vi "Dashboard Main.vi"() -> ()   [LabVIEW 2012]
uses:
  <vilib>/Utility/config.llb/Read Key (String).vi
  <vilib>/Utility/config.llb/Read Key (I32).vi
  <vilib>/Utility/config.llb/NI_LVConfig.lvlib
panel:
  in  "Y Coord":dbl=140.0
  in  "X Coord":dbl=200.0
  in  "Size":u16(ring)=1 items=["640x480", "320x240", "160x120"]
  in  "Compression":i32=30
  out "Mbps":dbl format="%#.1g"
  in  "Enable":bool=TRUE
  out "fps":dbl format="%#.1g"
  out "Camera Image":T1(plugin-control)
  out "Camera Image 2":T1(plugin-control)
  out "Camera IP 2":string
  out "Camera IP":string
  out "fps 2":dbl format="%#.1g"
  out "Mbps 2":dbl format="%#.1g"
  in  "Enable 2":bool=TRUE
  in  "Frame Rate":i32=15
  out "Battery Value":dbl(slide) scale=0.0..14.0 scale format="%#_2e"
  out "Battery":sgl(graph)
  out "Robot IP":string
  out "Mode":T2(ring)=enum."Auto Disabled"
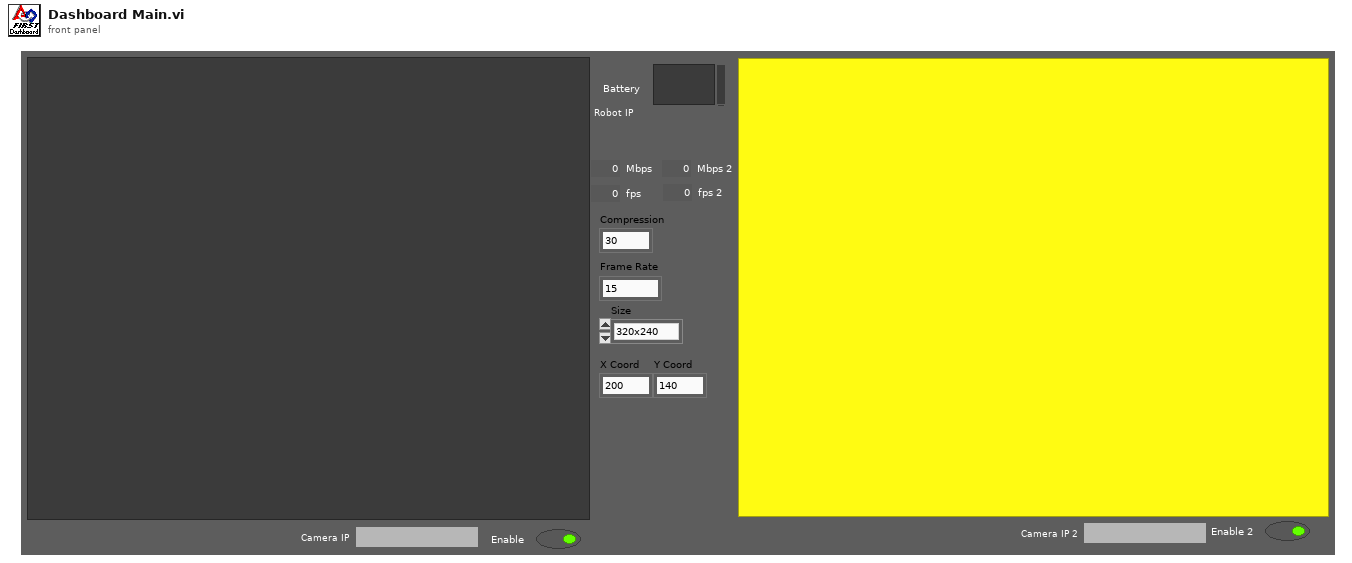
[diagram p1: front panel]
types:
  T1 = typedef "IMAQ Image.ctl" = refnum<image>
  T2 = enum8{"Tele-Op Disabled", "Tele-Op Enabled", "Auto Disabled", "Auto Enabled", "Test Disabled", "Test Enabled", ""}
  T3 = typedef "Image Type" = u32
  T4 = typedef "NI_LVConfig.lvlib/Config Data RefNum.ctl" = refnum<k1>
  T5 = cluster{"Competition mode":bool, "Robot Link":bool, "Autonomous":bool, "Enabled":bool, "E-Stop":bool, "Simulated":bool, "TestMode":bool, "Docked Window":bool}
  T6 = typedef "LVRectTypeDef.ctl" = cluster{"Left":i16, "Top":i16, "Right":i16, "Bottom":i16}
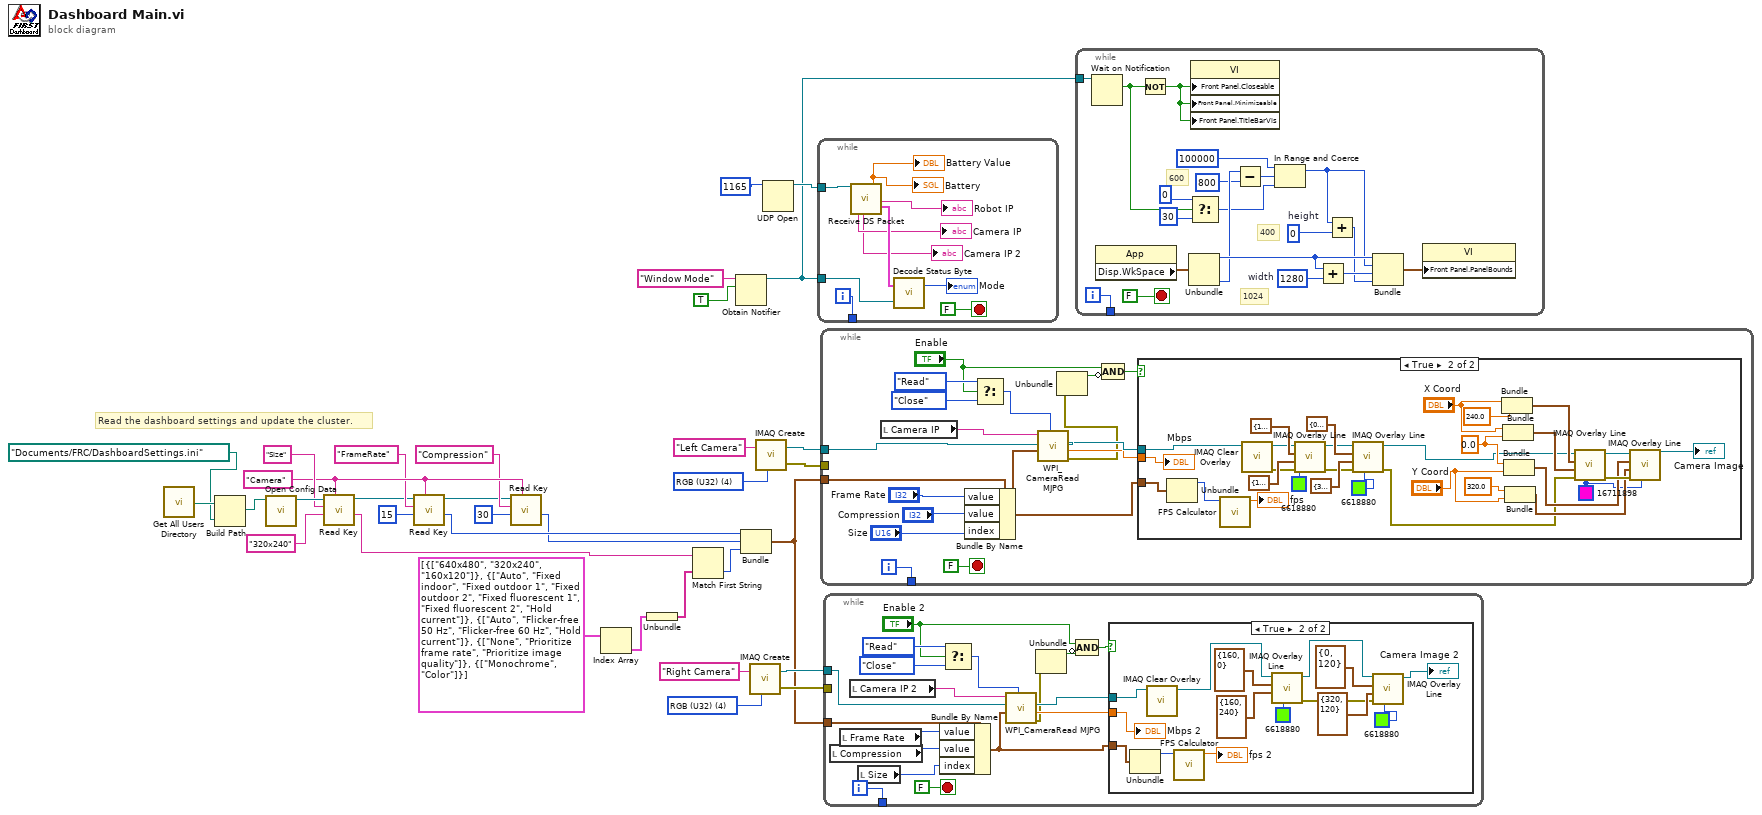
[diagram p0: block diagram]
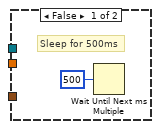
[diagram p2: hidden frame]
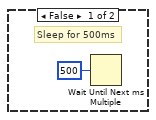
[diagram p3: hidden frame]
diagram:
  w4 = T3 4 items=["Grayscale (U8)", "Grayscale (I16)", "Grayscale (SGL)", "Complex (CSG)", "RGB (U32)", "HSL (U32)", "RGB (U64)"] ("Image Type")
  w20 = "Camera"
  w32 = T3 4 items=["Grayscale (U8)", "Grayscale (I16)", "Grayscale (SGL)", "Complex (CSG)", "RGB (U32)", "HSL (U32)", "RGB (U64)"] ("Image Type")
  # "Read the dashboard settings and update the cluster."
  n1 = call "Get All Users Directory.vi"() -> ("All User Path"=w25:path)
  n2 = Build Path(base path=w25, name or relative path=path "Documents/FRC/DashboardSettings.ini") -> (appended path=w24:path)
  n3 = call <vilib>:"Open Config Data.vi"("configuration file path"=w24) -> ("refnum"=w23:T4)  [unwired: 8 in, 2 out]
  n4 = call-poly <vilib>:"Read Key.vi"("section"=w20, "default value"="320x240", "key"="Size", "refnum"=w23) -> ("value"=w10:string, "refnum out"=w7:T4)  [unwired: 2 in, 4 out]
  n5 = call-poly <vilib>:"Read Key.vi"("section"=w20, "default value"=15, "key"="FrameRate", "refnum"=w7) -> ("value"=w15:i32, "refnum out"=w6:T4)  [unwired: 1 in, 5 out]
  n6 = call-poly <vilib>:"Read Key.vi"("section"=w20, "default value"=30, "key"="Compression", "refnum"=w6) -> ("value"=w14:i32)  [unwired: 1 in, 6 out]
  n7 = Index Array(array=cluster{string[]}[] [{["640x480", "320x240", "160x120"]}, {["Auto", "Fixed indoor", "Fixed outdoor 1", "Fixed outdoor 2", "Fixed fluorescent 1", "Fixed fluorescent 2", "Hold current"]}, {["Auto", "Flicker-free 50 Hz", "Flicker-free 60 Hz", "Hold current"]}, {["None", "Prioritize frame rate", "Prioritize image quality"]}, {["Monochrome", "Color"]}]) -> (element=w13:cluster{string[]})  [unwired: 1 in]
  n8 = Unbundle(w13) -> (w11:string[])
  n9 = Match First String(2:w11, 3:w10) -> (0:w9:i32)  [unwired: 1 out]
  n10 = Obtain Notifier(name (unnamed)="Window Mode", notification data type=TRUE) -> (notifier out=w26:refnum<notifier>)  [unwired: 2 in, 2 out]
  n11 = Bundle("value"=w15, "value"=w14, "index"=w9) -> (w1:cluster{"value":i32, "value":i32, "index":i32})  [unwired: 1 out]
  n12 = call "IMAQ Create"("Image Name"="Right Camera", "Image Type"=w4) -> ("New Image"=w3:T1, "error out"=w2:errorcluster)  [unwired: 2 in, 1 out]
  n13 = call "IMAQ Create"("Image Name"="Left Camera", "Image Type"=w32) -> ("New Image"=w30:T1, "error out"=w29:errorcluster)  [unwired: 2 in, 1 out]
  n14 = UDP Open(11:u16 1165 ("port")) -> (port=w33:refnum<k16>)  [unwired: 2 in, 4 out]
  n15 = while {
    tunnel: w33 -> [w42]
    tunnel: w26 -> [w40]
    tunnel: [w37] -> _
    i -> [w37]
    stop <- FALSE stop-if-true
    n16 = call "Receive DS Packet.vi"("Recv Socket"=w42) -> ("Camera IP Address"=→"Camera IP":string, "Camera IP Address 2"=→"Camera IP 2":string, "Battery"=→"Battery" →"Battery Value":sgl, "Robot IP Address"=→"Robot IP":string, "Status"=w43:T5)  [unwired: 8 in, 6 out]
    n17 = call "Decode Status Byte.vi"("Window Mode Notifier"=w40, "Status"=w43) -> ("Mode"=→"Mode":T2)  [unwired: 1 out]
  }
  n18 = while {
    tunnel: w30 -> [w59]
    tunnel: w29 -> [_]
    tunnel: [w61] -> _
    tunnel: w1 -> [w47]
    i -> [w61]
    stop <- FALSE stop-if-true
    n19 = local read "Camera IP"() -> (w60:string)
    n20 = Bundle By Name(cluster=w47, "value"="Frame Rate", "value"="Compression", "index"="Size") -> (w48:cluster{"value":i32, "value":i32, "index":i32})
    n21 = Select(t=enum16{"Read", "Reopen", "Close"}."Read" ("Operation"), s="Enable", f=enum16{"Read", "Reopen", "Close"}."Close" ("Operation")) -> (s? t:f=w54:enum16{"Read", "Reopen", "Close"})
    n22 = call <vilib>:"WPI_CameraRead MJPG.vi"("Operation"=w54, "Camera Settings"=w48, "Image"=w59, "address"=w60) -> ("error out"=w53:errorcluster, "Bandwidth (kbps)"=w57:dbl, "Image Out"=w58:T1)  [unwired: 5 in]
    n23 = Unbundle(w53) -> ("status"=w51:bool)  [unwired: 2 out]
    n24 = Compound Arithmetic op=AND("Enable", invert w51) -> (w50:bool)
    n25 = case shown="True" w50 {
      tunnel: w48 -> [_ w90]
      tunnel: w58 -> [_ w93]
      tunnel: w57 -> [_ w92]
      frame False {
        # "Sleep for 500ms"
        n26 = Wait Until Next ms Multiple(millisecond multiple=u32 500) -> ()  [unwired: 1 out]
      }
      frame True {
        w64 = u32 16711898 ("Color")
        w77 = 0.0 ("element")
        n27 = Unbundle(w90) -> ("value"=w81:i32)  [unwired: 2 out]
        n28 = call "FPS Calculator.vi"("Average Count"=w81) -> ("fps"=→"fps":dbl)  [unwired: 10 in]
        n29 = call "IMAQ Clear Overlay"("Image"=w93) -> ("error out"=w79:errorcluster, "Image Out"=w82:T1)  [unwired: 2 in, 7 out]
        n30 = call "IMAQ Overlay Line"("Color"=u32 6618880, "error in (no error)"=w79, "End Point"=cluster{"X":i32, "Y":i32} {"X"=160, "Y"=240}, "Start Point"=cluster{"X":i32, "Y":i32} {"X"=160, "Y"=0}, "Image"=w82) -> ("error out"=w87:errorcluster, "Image Out"=w86:T1)  [unwired: 5 in]
        n31 = call "IMAQ Overlay Line"("Color"=u32 6618880, "error in (no error)"=w87, "End Point"=cluster{"X":i32, "Y":i32} {"X"=320, "Y"=120}, "Start Point"=cluster{"X":i32, "Y":i32} {"X"=0, "Y"=120}, "Image"=w86) -> ("error out"=w65:errorcluster, "Image Out"=w66:T1)  [unwired: 5 in]
        n32 = Bundle("X Coord"="X Coord", "element"=240.0) -> (w70:cluster{"X Coord":dbl, "element":dbl})  [unwired: 1 in]
        n33 = Bundle("X Coord"="X Coord", "element"=w77) -> (w69:cluster{"X Coord":dbl, "element":dbl})  [unwired: 1 in]
        n34 = Bundle("element"=w77, "Y Coord"="Y Coord") -> (w68:cluster{"element":dbl, "Y Coord":dbl})  [unwired: 1 in]
        n35 = Bundle("element"=320.0, "Y Coord"="Y Coord") -> (w67:cluster{"element":dbl, "Y Coord":dbl})  [unwired: 1 in]
        n36 = call "IMAQ Overlay Line"("Color"=w64, "error in (no error)"=w65, "End Point"=w69, "Start Point"=w70, "Image"=w66) -> ("error out"=w72:errorcluster, "Image Out"=w73:T1)  [unwired: 5 in]
        n37 = call "IMAQ Overlay Line"("Color"=w64, "error in (no error)"=w72, "End Point"=w67, "Start Point"=w68, "Image"=w73) -> ("Image Out"=→"Camera Image":T1)  [unwired: 5 in, 1 out]
        "Mbps" <- w92
      }
    }
  }
  n38 = while {
    tunnel: w3 -> [w108]
    tunnel: [w110] -> _
    tunnel: w2 -> [_]
    tunnel: w1 -> [w96]
    i -> [w110]
    stop <- FALSE stop-if-true
    n39 = local read "Compression"() -> (w95:i32)
    n40 = local read "Frame Rate"() -> (w98:i32)
    n41 = local read "Camera IP 2"() -> (w109:string)
    n42 = local read "Size"() -> (w94:u16)
    n43 = Bundle By Name(cluster=w96, "value"=w98, "value"=w95, "index"=w94) -> (w97:cluster{"value":i32, "value":i32, "index":i32})
    n44 = Select(t=enum16{"Read", "Reopen", "Close"}."Read" ("Operation"), s="Enable 2", f=enum16{"Read", "Reopen", "Close"}."Close" ("Operation")) -> (s? t:f=w103:enum16{"Read", "Reopen", "Close"})
    n45 = call <vilib>:"WPI_CameraRead MJPG.vi"("Operation"=w103, "Camera Settings"=w97, "Image"=w108, "address"=w109) -> ("error out"=w102:errorcluster, "Bandwidth (kbps)"=w106:dbl, "Image Out"=w107:T1)  [unwired: 5 in]
    n46 = Unbundle(w102) -> ("status"=w100:bool)  [unwired: 2 out]
    n47 = Compound Arithmetic op=AND("Enable 2", invert w100) -> (w99:bool)
    n48 = case shown="True" w99 {
      tunnel: w97 -> [_ w124]
      tunnel: w107 -> [_ w127]
      tunnel: w106 -> [_ w126]
      frame False {
        # "Sleep for 500ms"
        n49 = Wait Until Next ms Multiple(millisecond multiple=u32 500) -> ()  [unwired: 1 out]
      }
      frame True {
        n50 = Unbundle(w124) -> ("value"=w123:i32)  [unwired: 2 out]
        n51 = call "IMAQ Clear Overlay"("Image"=w127) -> ("Image Out"=w114:T1)  [unwired: 2 in, 8 out]
        n52 = call "FPS Calculator.vi"("Average Count"=w123) -> ("fps"=→"fps 2":dbl)  [unwired: 10 in]
        n53 = call "IMAQ Overlay Line"("Color"=u32 6618880, "End Point"=cluster{"X":i32, "Y":i32} {"X"=160, "Y"=240}, "Start Point"=cluster{"X":i32, "Y":i32} {"X"=160, "Y"=0}, "Image"=w114) -> ("error out"=w120:errorcluster, "Image Out"=w119:T1)  [unwired: 6 in]
        n54 = call "IMAQ Overlay Line"("Color"=u32 6618880, "error in (no error)"=w120, "End Point"=cluster{"X":i32, "Y":i32} {"X"=320, "Y"=120}, "Start Point"=cluster{"X":i32, "Y":i32} {"X"=0, "Y"=120}, "Image"=w119) -> ("Image Out"=→"Camera Image 2":T1)  [unwired: 5 in, 1 out]
        "Mbps 2" <- w126
      }
    }
  }
  n55 = while {
    tunnel: w26 -> [w146]
    tunnel: [w144] -> _
    i -> [w144]
    stop <- FALSE stop-if-true
    w136 = 1280  # width
    w139 = 0  # height
    # "600"
    # "1024"
    # "400"
    n56 = Wait on Notification(notifier=w146) -> (notification=w131:bool)  [unwired: 3 in, 3 out]
    n57 = property class="App"() -> ("Disp.WkSpace"=w142:T6)  [unwired: 2 in, 2 out]
    n58 = Not(x=w131) -> (.not. x?=w145:bool)
    n59 = Unbundle(w142) -> ("Left"=w140:i16, "Bottom"=w137:i16)  [unwired: 2 out]
    n60 = Select(t=0, s=w131, f=30) -> (s? t:f=w130:i32)
    n61 = property class="VI"("Front Panel.Closeable"=w145, "Front Panel.Minimizeable"=w145, "Front Panel.TitleBarVis"=w145) -> ()  [unwired: 2 in, 2 out]
    n62 = Subtract(x=w137, y=800) -> (x-y=w134:i32)
    n63 = In Range and Coerce(upper limit=100000, x=w134, lower limit=w130) -> (coerced(x)=w128:i32)  [unwired: 1 out]
    n64 = Add(x=w140, y=w136) -> (x+y=w141:i32)
    n65 = Add(x=w128, y=w139) -> (x+y=w138:i32)
    n66 = Bundle("Left"=w140, w128, w141, w138) -> (w143:cluster{"Left":i16, i32, i32, i32})  [unwired: 1 out]
    n67 = property class="VI"("Front Panel.PanelBounds"=w143) -> ()  [unwired: 2 in, 2 out]
  }
